vi "Set Magnet.vi"(4 "Mode":T2, 6 "Axis":T1, 8 "error in (no error)":errorcluster, 9 "Target Rate (T/min)":dbl, 10 "Target Field (T)":dbl, 11 "Instrument.Cryostat in":refnum<class "Instrument.Cryostat.lvclass">) -> (0 "error out":errorcluster, 3 "Instrument.Cryostat out":refnum<class "Instrument.Cryostat.lvclass">)   [LabVIEW 2019, in "Instrument.Cryostat.lvclass"]
uses:
  Instrument.Cryostat.lvclass
  Typedefs/Magnet Mode--Enum.ctl
  Typedefs/Magnet Axis--Enum.ctl
  Typedefs/Set Magnet--cluster.ctl
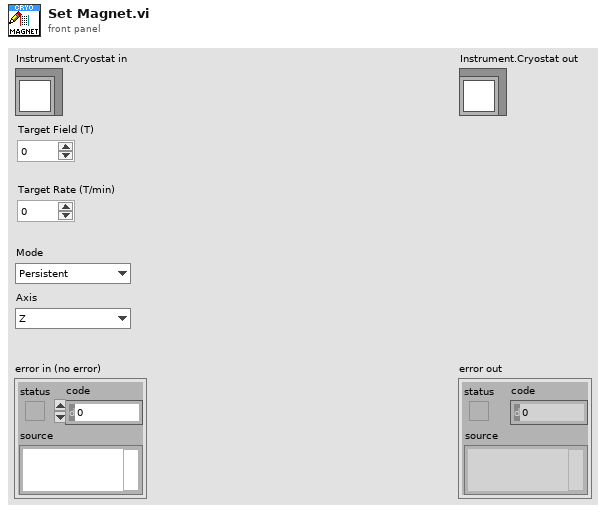
[diagram p1: front panel]
types:
  T1 = typedef "Instrument.Cryostat.lvclass/Magnet Axis--Enum.ctl" = enum16{"Z", "X", "Y"}
  T2 = typedef "Instrument.Cryostat.lvclass/Magnet Mode--Enum.ctl" = enum16{"Persistent", "Driven"}
  T3 = typedef "Instrument.Cryostat.lvclass/Set Magnet--cluster.ctl" = cluster{"Field (T)":dbl, "Rate (T/min)":dbl, "Axis":T1, "Mode":T2}
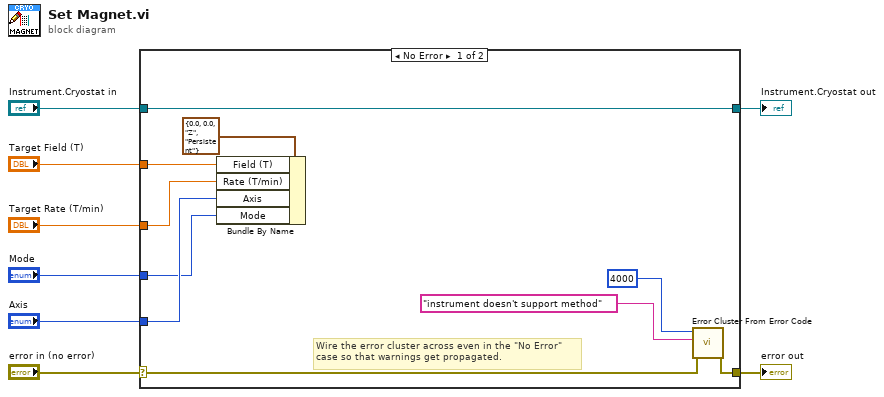
[diagram p0: block diagram]
diagram:
  n1 = case shown="No Error" "error in (no error)" {
    selector: "error in (no error)" -> [w15 w20]
    tunnel: [w14 w20] -> w7
    tunnel: [w18 w19] -> w5
    tunnel: "Instrument.Cryostat in" -> [w18 w19]
    tunnel: "Target Field (T)" -> [w12 _]
    tunnel: "Target Rate (T/min)" -> [w11 _]
    tunnel: "Axis" -> [w10 _]
    tunnel: "Mode" -> [w9 _]
    frame No Error {
      # "Wire the error cluster across even in the \"No Error\"\ncase so that warnings get propagated."
      n2 = Bundle By Name(cluster=T3 {"Field (T)"=0.0, "Rate (T/min)"=0.0, "Axis"=enum."Z", "Mode"=enum."Persistent"} ("Set Magnet Field"), "Field (T)"=w12, "Rate (T/min)"=w11, "Axis"=w10, "Mode"=w9) -> ()  [unwired: 1 out]
      n3 = call <vilib>:"Error Cluster From Error Code.vi"("error in (no error)"=w15, "error message (\"\")"="instrument doesn't support method" ("error message (\"\")"), "error code (0)"=4000) -> ("error out"=w14:errorcluster)  [unwired: 6 in]
    }
    frame Error {
    }
  }
  "error out" <- w7
  "Instrument.Cryostat out" <- w5
